vi "Hash string to byte array.vi"(11 "String to Encode":string) -> (3 "H Array":u32[](array[numeric]) format="%08x")   [LabVIEW 2019]
doc: "Takes a string buffer and creates a 8 x 32 bit word hash using the SHA-256 algorithm."
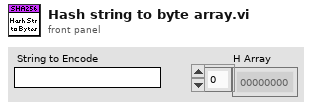
[diagram p1: front panel]
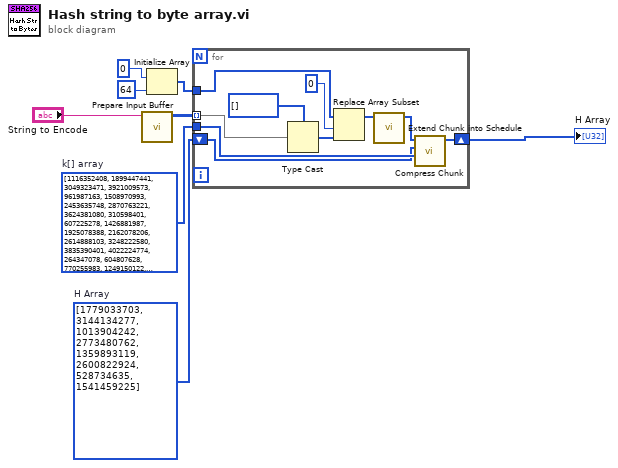
[diagram p0: block diagram]
diagram:
  w8 = u32[] [1116352408, 1899447441, 3049323471, 3921009573, 961987163, 1508970993, 2453635748, 2870763221, 3624381080, 310598401, 607225278, 1426881987, 1925078388, 2162078206, 2614888103, 3248222580, 3835390401, 4022224774, 264347078, 604807628, 770255983, 1249150122, 1555081692, 1996064986, 2554220882, 2821834349, 2952996808, 3210313671, 3336571891, 3584528711, 113926993, 338241895, 666307205, 773529912, 1294757372, 1396182291, 1695183700, 1986661051, 2177026350, 2456956037, 2730485921, 2820302411, 3259730800, 3345764771, 3516065817, 3600352804, 4094571909, 275423344, 430227734, 506948616, 659060556, 883997877, 958139571, 1322822218, 1537002063, 1747873779, 1955562222, 2024104815, 2227730452, 2361852424, 2428436474, 2756734187, 3204031479, 3329325298]  # k[] array
  w7 = u32[] [1779033703, 3144134277, 1013904242, 2773480762, 1359893119, 2600822924, 528734635, 1541459225]  # H Array
  n1 = call "Prepare Input Buffer.vi"("String to Encode"="String to Encode") -> ("Chunked MEssage"=w3:u8[][])  [unwired: 10 in]
  n2 = Initialize Array(u32 0 ("element"), 64 ("dimension size")) -> (w6:u32[])
  n3 = for {
    tunnel: w3 -> [w18] mode=indexing
    tunnel: w6 -> [w16]
    tunnel: w8 -> [w11]
    shift-right: [w9] -> w2
    shift-left: w7 -> [w10]
    n4 = Type Cast(type=u32[] [], x=w18) -> (*(type *) &x=w15:u32[])
    n5 = Replace Array Subset(array=w16, new element=w15, index=0) -> (w13:u32[])
    n6 = call "Extend Chunk into Schedule.vi"("Array in"=w13) -> ("Array out"=w12:u32[])  [unwired: 10 in]
    n7 = call "Compress Chunk.vi"("Key Array"=w11, "Hash In"=w10, "Data Array In"=w12) -> ("Hash Out"=w9:u32[])  [unwired: 8 in]
  }
  "H Array" <- w2
